vi "moj global.vi"() -> ()   [LabVIEW 2015]
panel:
  out "Cluster":T1
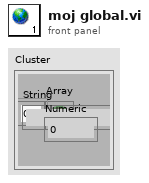
[diagram p1: front panel]
types:
  T1 = cluster{"Array":bool[], "String":string, "Numeric":dbl}
diagram:
